vi "Save.vi"(8 "Error In":errorcluster, 11 "VISA resource name":refnum<visa-resource-name>) -> (0 "Error Out":errorcluster, 3 "VISA resource name out":refnum<visa-resource-name>)   [LabVIEW 2013]
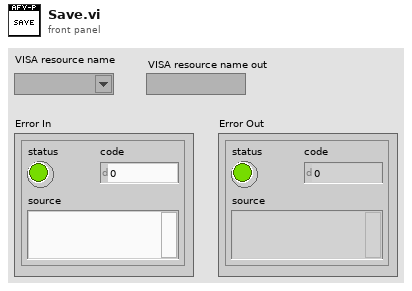
[diagram p1: front panel]
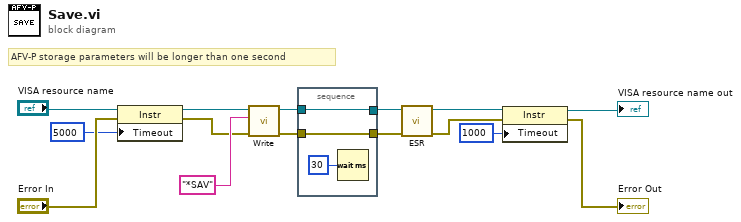
[diagram p0: block diagram]
diagram:
  # "AFV-P storage parameters will be longer than one second"
  n1 = property class="Instr"(reference="VISA resource name", error in="Error In", "Timeout"=u32 5000 ("General Settings:Timeout Value")) -> (reference out=w8:refnum<visa-resource-name>, error out=w10:errorcluster)
  n2 = call "Write.vi"("Error In"=w10, "Write Buffer"="*SAV", "VISA resource name"=w8) -> ("Error Out"=w14:errorcluster, "VISA resource name out"=w15:refnum<visa-resource-name>)  [unwired: 7 in]
  n3 = stacked-sequence {
    tunnel: [w17] -> w7
    tunnel: w15 -> [w17]
    tunnel: [w16] -> w6
    tunnel: w14 -> [w16]
    frame #0 {
      n4 = Wait (ms)(milliseconds to wait=u32 30) -> ()  [unwired: 1 out]
    }
  }
  n5 = call "ESR.vi"("Error In"=w6, "VISA resource name"=w7) -> ("Error Out"=w3:errorcluster, "VISA resource name out"=w5:refnum<visa-resource-name>)  [unwired: 8 in]
  n6 = property class="Instr"(reference=w5, error in=w3, "Timeout"=u32 1000 ("General Settings:Timeout Value")) -> (reference out=→"VISA resource name out":refnum<visa-resource-name>, error out=→"Error Out":errorcluster)
